vi "instrument_error_query.vi"(5 "Beginning error message string (\"\")":string, 7 "Add instrument error to error cluster (T)":bool=TRUE, 8 "error in":errorcluster, 10 "Query (SYST:ERR?)":string="SYST:ERR?", 11 "VISA resource name":refnum<visa-resource-name>) -> (0 "error out":errorcluster, 1 "Error Message(s) out":string, 2 "Error Code":i32, 3 "VISA resource name out":refnum<visa-resource-name>)   [LabVIEW 2014, in "rszvl_rsidr_core.lvlib"]
uses:
  rszvl_rsidr_core.lvlib
  type_Error_Codes.ctl
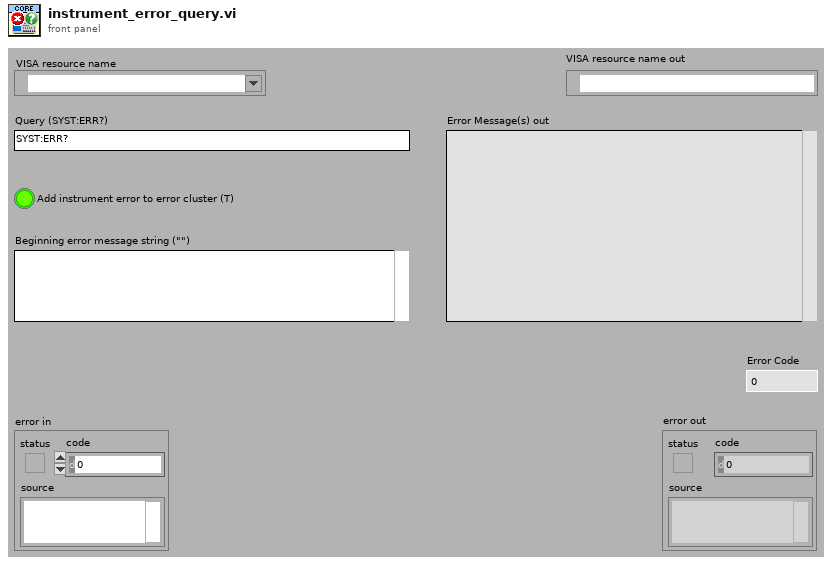
[diagram p1: front panel]
types:
  T1 = typedef "rszvl_rsidr_core.lvlib/type_Error_Codes.ctl" = enum16{"No_error", "VISA_err_ResourceNotFound", "VISA_err_Timeout", "VISA_warn_MoreDataAvailable", "RS_err_MissingCallback", "RS_err_InvalidAttribute", "RS_err_InvalidValue", "RS_err_UnknownResource", "RS_err_AlreadyInitialized", "RS_err_InstrumentStatus", "RS_err_BadRepCapName", "RS_err_TypesMismatch", "RS_err_ValueNotSupported", "RS_err_InvalidRngTable", "RS_err_IDqueryFail", "RS_err_UnexpResponse", "VISA_warn_ConfigNotLoaded", "RS_err_AttributeNotReadable", "RS_err_AttributeNotWritable", "RS_err_InstrumentType", "RS_err_InstrumentOption", "VISA_err_InvalidSize", "RS_err_ReliabilityIndicator", "VISA_warn_UnknownStatus", "VISA_warn_TermCharRead", "VISA_err_IO_error"}
  T2 = typedef "rszvl_rsidr_core.lvlib/type_Session_Data.ctl" = cluster{"Instr type":string, "Instr type for err. msg.":string, "Installed Options":string[], "OPC Timeout":i32, "Query Instrument Status":bool, "Check Range":bool, "Check Options":bool, "Add LF to Write":bool, "Simulate":bool, "Logging":bool, "Logging params":variant, "Interface Type":enum16{"Unknown", "GPIB", "VXI", "GPIB_VXI", "ASRL", "PXI", "TCPIP", "USB", "SOCKET"}, "Fast Sweep":i32, "AdditionalFlags":i32, "WaitBeforeWrite":i32, "WaitBeforeRead":i32, "BinDataChunkSize":i64}
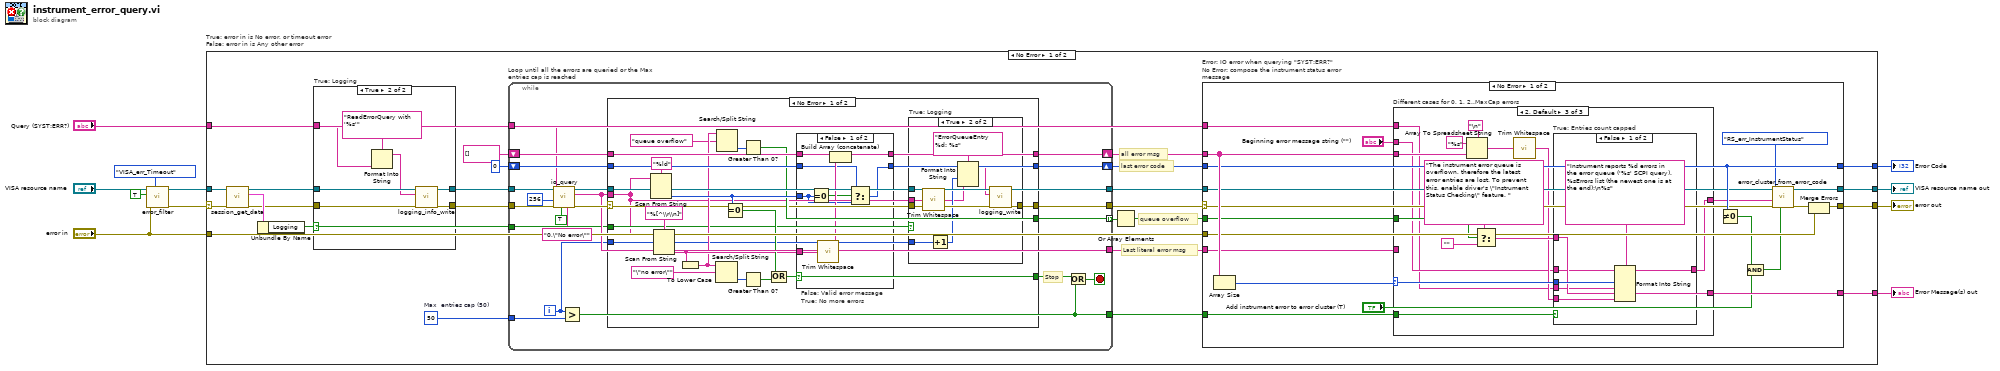
[diagram p0: block diagram]
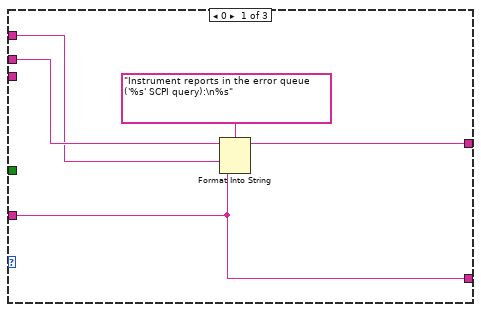
[diagram p3: hidden frame]
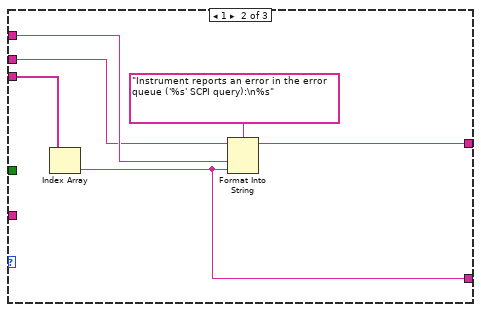
[diagram p4: hidden frame]
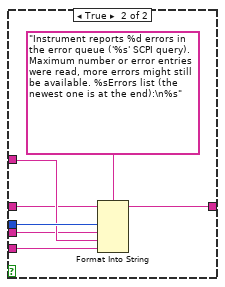
[diagram p5: hidden frame]
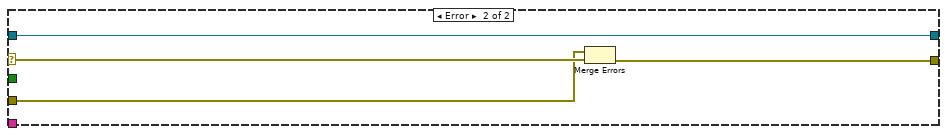
[diagram p6: hidden frame]
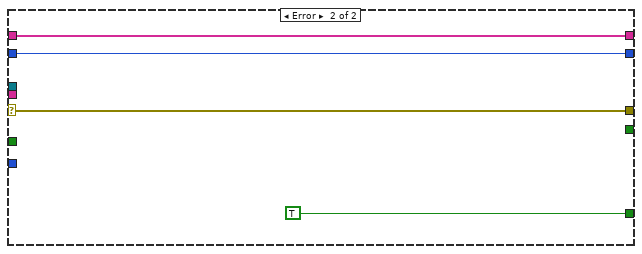
[diagram p9: hidden frame]
diagram:
  n1 = call "error_filter.vi"("Error Enum in"=type_Error_Codes."VISA_err_Timeout" ("Code to detect"), "error in"="error in", "Clear detected code (F)"=TRUE ("Clear detected error (F)"), "VISA resource name"="VISA resource name") -> ("error out"=w5:errorcluster, "VISA resource name out"=w2:refnum<visa-resource-name>)  [unwired: 5 in, 1 out]
  n2 = case "True: error in is No error, or timeout error\nFalse: error in is Any other error" shown="No Error" w5 {
    selector: w5 -> [w20 _]
    tunnel: [w29 _] -> w9
    tunnel: [w31 _] -> w11
    tunnel: [w15 w178] -> w8
    tunnel: w2 -> [w21 w178]
    tunnel: "error in" -> [w24 w177]
    tunnel: [w23 w177] -> w10
    tunnel: "Query (SYST:ERR?)" -> [w12 _]
    frame No Error {
      w28 = 50  # Max  entries cap (50)
      # "queue overflow"
      # "Last literal error msg"
      # "last error code"
      # "all error msg"
      n3 = call "session_get_data.vi"("error in"=w20, "VISA resource name"=w21) -> ("error out"=w17:errorcluster, "Session User Data out"=w19:T2, "VISA resource name out"=w18:refnum<visa-resource-name>)  [unwired: 7 in]
      n4 = Unbundle By Name(w19) -> ("Logging"=w16:bool)
      n5 = case "True: Logging" shown="True" w16 {
        tunnel: w18 -> [w38 w45]
        tunnel: [w38 w44] -> w14
        tunnel: w17 -> [w37 w43]
        tunnel: [w37 w42] -> w13
        tunnel: w12 -> [_ w40]
        frame False {
        }
        frame True {
          n6 = Format Into String(format string="ReadErrorQuery with '%s'" ("String to write"), w40) -> (resulting string=w39:string)  [unwired: 2 in, 1 out]
          n7 = call "logging_info_write.vi"("error in"=w43, "String to write"=w39, "VISA resource name"=w45) -> ("error out"=w42:errorcluster, "VISA resource name out"=w44:refnum<visa-resource-name>)  [unwired: 7 in]
        }
      }
      n8 = while "Loop until all the errors are queried or the Max  entries cap is reached" {
        tunnel: [w115] -> w22
        tunnel: w14 -> [w116]
        tunnel: [w114] -> w32
        shift-right: [w128] -> w34
        shift-left: string[] [] -> [w129]
        shift-right: [w126] -> w33
        shift-left: 0 -> [w127]
        tunnel: [w118] -> w30
        tunnel: w28 -> [w123]
        tunnel: [w122] -> w27
        tunnel: [w121] -> w26 mode=indexing
        tunnel: w13 -> [w117]
        tunnel: w16 -> [w113]
        tunnel: w12 -> [w109]
        i -> [w112]
        stop <- w124 stop-if-true
        # "Stop"
        n9 = call "io_query.vi"("Simulation read buffer (\"Simulation\")"="0,\"No error\"" ("Simulation read buffer \n(\"Simulation\")"), "Block Logging (F)"=TRUE, "error in"=w117, "Bytes to read (2048)"=u32 256 ("Bytes"), "write buffer"=w109, "VISA resource name"=w116) -> ("error out"=w120:errorcluster, "read buffer"=w118:string, "VISA resource name out"=w115:refnum<visa-resource-name>)  [unwired: 2 in, 1 out]
        n10 = Greater?(x=w112, y=w123) -> (0:w122:bool)
        n11 = case shown="No Error" w120 {
          selector: w120 -> [w135 w173]
          tunnel: [w146 TRUE] -> w125
          tunnel: w129 -> [w145 w176]
          tunnel: [w144 w176] -> w128
          tunnel: w127 -> [w141 w175]
          tunnel: [w140 w175] -> w126
          tunnel: [w136 _] -> w121
          tunnel: w118 -> [w130 _]
          tunnel: w115 -> [w134 _]
          tunnel: [w133 w173] -> w114
          tunnel: w113 -> [w132 _]
          tunnel: w112 -> [w131 _]
          frame No Error {
            n12 = Scan From String(format string="%ld", input string=w130) -> (output 1=w142:i32)  [unwired: 3 in, 3 out]
            n13 = Scan From String(format string="%[^\\r\\n]", input string=w130) -> (output 1=w143:string)  [unwired: 3 in, 3 out]
            n14 = To Lower Case(string=w143) -> (all lower case string=w139:string)
            n15 = Search/Split String(string=w139, search string/char (-)="\"no error\"") -> (offset of match=w149:i32)  [unwired: 1 in, 2 out]
            n16 = Search/Split String(string=w139, search string/char (-)="queue overflow") -> (offset of match=w137:i32)  [unwired: 1 in, 2 out]
            n17 = Equal To 0?(x=w142) -> (x = 0?=w148:bool)
            n18 = Greater Than 0?(x=w137) -> (x > 0?=w136:bool)
            n19 = Greater Than 0?(x=w149) -> (x > 0?=w147:bool)
            n20 = Compound Arithmetic op=OR(w148, w147) -> (w146:bool)
            n21 = case "False: Valid error message\nTrue: No more errors" shown="False" w146 {
              tunnel: w145 -> [w169 w172]
              tunnel: [w170 w172] -> w144
              tunnel: w143 -> [w168 _]
              tunnel: w142 -> [w163 _]
              tunnel: w141 -> [w165 w171]
              tunnel: [w164 w171] -> w140
              frame False {
                n22 = Equal To 0?(x=w163) -> (x = 0?=w166:bool)
                n23 = call "Trim Whitespace.vi"("string"=w168) -> ("trimmed string"=w167:string)  [unwired: 1 in]
                n24 = Build Array (concatenate)(w169, w167) -> (w170:string[])
                n25 = Select(t=w165, s=w166, f=w163) -> (s? t:f=w164:i32)
              }
              frame True {
              }
            }
            n26 = case "True: Logging" shown="True" w132 {
              tunnel: w135 -> [w153 w162]
              tunnel: w134 -> [_ w161]
              tunnel: [w153 w160] -> w133
              tunnel: w131 -> [_ w157]
              tunnel: w130 -> [_ w155]
              frame False {
              }
              frame True {
                n27 = call "Trim Whitespace.vi"("string"=w155) -> ("trimmed string"=w154:string)  [unwired: 1 in]
                n28 = Increment(x=w157) -> (x+1=w156:i32)
                n29 = Format Into String(format string="ErrorQueueEntry %d: %s", w156, w154) -> (resulting string=w159:string)  [unwired: 2 in, 1 out]
                n30 = call "logging_write.vi"("error in"=w162, "String to write"=w159, "VISA resource name"=w161) -> ("error out"=w160:errorcluster)  [unwired: 7 in, 1 out]
              }
            }
          }
          frame Error {
          }
        }
        n31 = Or(x=w125, y=w122) -> (x .or. y?=w124:bool)
      }
      n32 = Or Array Elements(Boolean array=w26) -> (logical OR=w25:bool)
      n33 = case "Error: IO error when querying \"SYST:ERR?\"\nNo Error: compose the instrument status error message" shown="No Error" w32 {
        selector: w32 -> [w52 w108]
        tunnel: [w58 w106] -> w23
        tunnel: [w62 _] -> w29
        tunnel: [w56 _] -> w31
        tunnel: w34 -> [w64 _]
        tunnel: w33 -> [w56 _]
        tunnel: w30 -> [w63 _]
        tunnel: w27 -> [w61 _]
        tunnel: w25 -> [w60 _]
        tunnel: w24 -> [w57 w107]
        tunnel: w22 -> [w51 w105]
        tunnel: [w55 w105] -> w15
        tunnel: w12 -> [w46 _]
        frame No Error {
          n34 = Array Size(array=w64) -> (size(s)=w65:i32)
          n35 = case "Different cases for 0, 1, 2..MaxCap errors" shown="2, Default" w65 {
            selector: w65 -> [_ _ w88]
            tunnel: [w67 w75 w89] -> w53
            tunnel: w64 -> [_ w71 w90]
            tunnel: w63 -> [w66 _ _]
            tunnel: [w66 w72 w79] -> w62
            tunnel: w61 -> [_ _ w84]
            tunnel: w60 -> [_ _ w83]
            tunnel: "Beginning error message string (\"\")" -> [w69 w73 w78]
            tunnel: w46 -> [w68 w74 w77]
            frame 0 {
              n36 = Format Into String(format string="Instrument reports in the error queue ('%s' SCPI query):\n%s" ("Source"), initial string=w69, w68, w66) -> (resulting string=w67:string)  [unwired: 1 in, 1 out]
            }
            frame 1 {
              n37 = Index Array(array=w71) -> (element=w72:string)  [unwired: 1 in]
              n38 = Format Into String(format string="Instrument reports an error in the error queue ('%s' SCPI query):\n%s" ("Source"), initial string=w73, w74, w72) -> (resulting string=w75:string)  [unwired: 1 in, 1 out]
            }
            frame 2, Default {
              n39 = Array To Spreadsheet String(delimiter (Tab)="\n" ("Line Feed Constant"), array=w90, 3:"%s" ("format string")) -> (spreadsheet string=w85:string)
              n40 = Select(t="The instrument error queue is overflown, therefore the latest error entries are lost. To prevent this, enable driver's \"Instrument Status Checking\" feature. " ("Source"), s=w83, f="" ("Empty String Constant")) -> (s? t:f=w80:string)
              n41 = call "Trim Whitespace.vi"("string"=w85) -> ("trimmed string"=w79:string)  [unwired: 1 in]
              n42 = case "True: Entries count capped" shown="False" w84 {
                tunnel: [w96 w103] -> w89
                tunnel: w88 -> [w95 w102]
                tunnel: w79 -> [w94 w101]
                tunnel: w80 -> [w93 w100]
                tunnel: w78 -> [w92 w99]
                tunnel: w77 -> [w91 w98]
                frame False {
                  n43 = Format Into String(format string="Instrument reports %d errors in the error queue ('%s' SCPI query). %sErrors list (the newest one is at the end):\n%s" ("Source"), initial string=w92, w95, w91, w93, w94) -> (resulting string=w96:string)  [unwired: 1 in, 1 out]
                }
                frame True {
                  n44 = Format Into String(format string="Instrument reports %d errors in the error queue ('%s' SCPI query). Maximum number or error entries were read, more errors might still be available. %sErrors list (the newest one is at the end):\n%s" ("Source"), initial string=w99, w102, w98, w100, w101) -> (resulting string=w103:string)  [unwired: 1 in, 1 out]
                }
              }
            }
          }
          n45 = Not Equal To 0?(x=w56) -> (x != 0?=w50:bool)
          n46 = Compound Arithmetic op=AND(w50, "Add instrument error to error cluster (T)") -> (w48:bool)
          n47 = call "error_cluster_from_error_code.vi"("error creation enabled (T)"=w48, "error in"=w52, "error message (\"\")"=w53, "Error Enum in"=type_Error_Codes."RS_err_InstrumentStatus", "VISA resource name"=w51) -> ("error out"=w59:errorcluster, "VISA resource name out"=w55:refnum<visa-resource-name>)  [unwired: 5 in]
          n48 = Merge Errors(w59, w57) -> (w58:errorcluster)
        }
        frame Error {
          n49 = Merge Errors(w107, w108) -> (w106:errorcluster)
        }
      }
    }
    frame Error {
    }
  }
  "Error Message(s) out" <- w9
  "Error Code" <- w11
  "VISA resource name out" <- w8
  "error out" <- w10
